vi "Autonomous Independent(2).vi"() -> ()   [LabVIEW 2014]
doc: "This VI is called when autonomous begins, and will automatically be terminated when autonomous ends. You can carry out timed or sensor driven robot movement independently without needing to return to the caller."
uses:
  <vilib>/Rock Robotics/WPI/Joystick/WPI_JoystickGetSetRefNum.vi
  <vilib>/Rock Robotics/Network Tables/SD Write Numeric Array.vi
  <vilib>/Rock Robotics/Network Tables/SD Read Number.vi
  <vilib>/Rock Robotics/WPI/RobotDrive/WPI_RobotDriveGetSetRefNum.vi
  <vilib>/Rock Robotics/WPI/RobotDrive/WPI_RobotDriveMecanumDrive_Cartesian.vi
  Robot Global Data.vi
panel:
  out "Current Movement, for debugging":T1 {"Z Joystick Value" scale=-1.0..1.0; "Y Joystick Value" scale=1.0..-1.0; "X Joystick Value" scale=-1.0..1.0}
  in  "Array of robot movements":T2(array[cluster]) {"Z Joystick Value" scale=-1.0..1.0; "Y Joystick Value" scale=1.0..-1.0; "X Joystick Value" scale=-1.0..1.0}
  # "Be sure to right-click and choose Data Operations>>Make Current Value default if you want to save the array values with the VI"
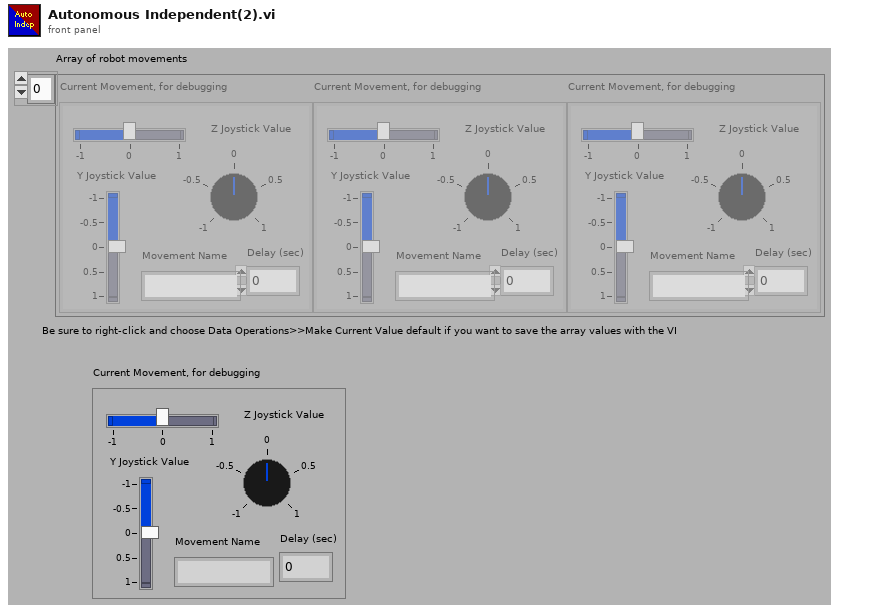
[diagram p1: front panel]
types:
  T1 = cluster{"X Joystick Value":dbl, "Y Joystick Value":dbl, "Z Joystick Value":dbl, "Delay (sec)":dbl, "Movement Name":string}
  T2 = cluster{"X Joystick Value":dbl, "Y Joystick Value":dbl, "Z Joystick Value":dbl, "Delay (sec)":dbl, "Movement Name":string}[]
  T3 = typedef "WPI_JoystickDevRef.ctl" = cluster{"Device":T4}
  T4 = typedef "WPI_JoystickDeviceEnum.ctl" = enum16{"USB 0", "USB 1", "USB 2", "USB 3", "USB 4", "USB 5"}
  T5 = typedef "WPI_EncoderDevRef.ctl" = cluster{"DevStatus":errorcluster, "EncoderIndex":T6, "CounterIndex":T7, "DistancePerCount":dbl, "Decoding Type":T8}
  T6 = typedef "FPGA_EncoderIdx.ctl" = enum8{"Enc 0", "Enc 1", "Enc 2", "Enc 3", "Enc 4", "Enc 5", "Enc 6", "Enc 7", "Invalid"}
  T7 = typedef "FPGA_CounterCtrSystemIndex.ctl" = enum8{"Ctr 0", "Ctr 1", "Ctr 2", "Ctr 3", "Ctr 4", "Ctr 5", "Ctr 6", "Ctr 7", "Invalid"}
  T8 = typedef "WPI_EncoderType.ctl" = enum16{"1x", "2x", "4x"}
  T9 = typedef "WPI_MotorControlDeviceRef.ctl" = cluster{"DeviceStatus":errorcluster, "Type":T10, "PWM":cluster{"Controller":T11, "PWM Channel":T12, "DeadBand":T13}, "CAN":cluster{"Device Number":u8, "Control Mode":T14, "Semaphore":T15, "Max Vout":dbl, "TalonSRX Control Mode":T16}, "Invert":bool, "TransformRef":T17, "InvTransformRef":T17}
  T10 = typedef "WPI_MotorControlType.ctl" = enum16{"PWM", "CAN", "CANTalonSRX"}
  T11 = typedef "FPGA_TypedefDigitalModule.ctl" = enum16{"Controller 1"}
  T12 = typedef "FPGA_DIOPWMChannel.ctl" = enum8{"PWM 0", "PWM 1", "PWM 2", "PWM 3", "PWM 4", "PWM 5", "PWM 6", "PWM 7", "PWM 8", "PWM 9", "PWM MXP 0", "PWM MXP 1", "PWM MXP 2", "PWM MXP 3", "PWM MXP 4", "PWM MXP 5", "PWM MXP 6", "PWM MXP 7", "PWM MXP 8", "PWM MXP 9", "Invalid"}
  T13 = typedef "WPI_PWMDeadband.ctl" = cluster{"Name":string, "maxPositivePwm":i32, "minPositivePwm":i32, "centerPwm":i32, "maxNegativePwm":i32, "minNegativePwm":i32, "angularRange":u16}
  T14 = typedef "WPI_CANJaguar_ControlMode.ctl" = enum8{"Percent VBus", "Current", "Speed", "Position", "Voltage"}
  T15 = typedef "Semaphore RefNum" = refnum<k1>
  T16 = typedef "WPI_CANTalonSRX_APIControlMode.ctl" = enum8{"Percent VBus", "Speed", "Position", "Slave", "Unchanged / Invalid"}
  T17 = typedef "WPI_PWMTransform_ConPane.ctl" = refnum<vi>
  T18 = typedef "WPI_RobotDriveDevRef.ctl" = cluster{"DevStatus":errorcluster, "Motors[]":T9[], "Square Inputs":bool, "Max Output":dbl}
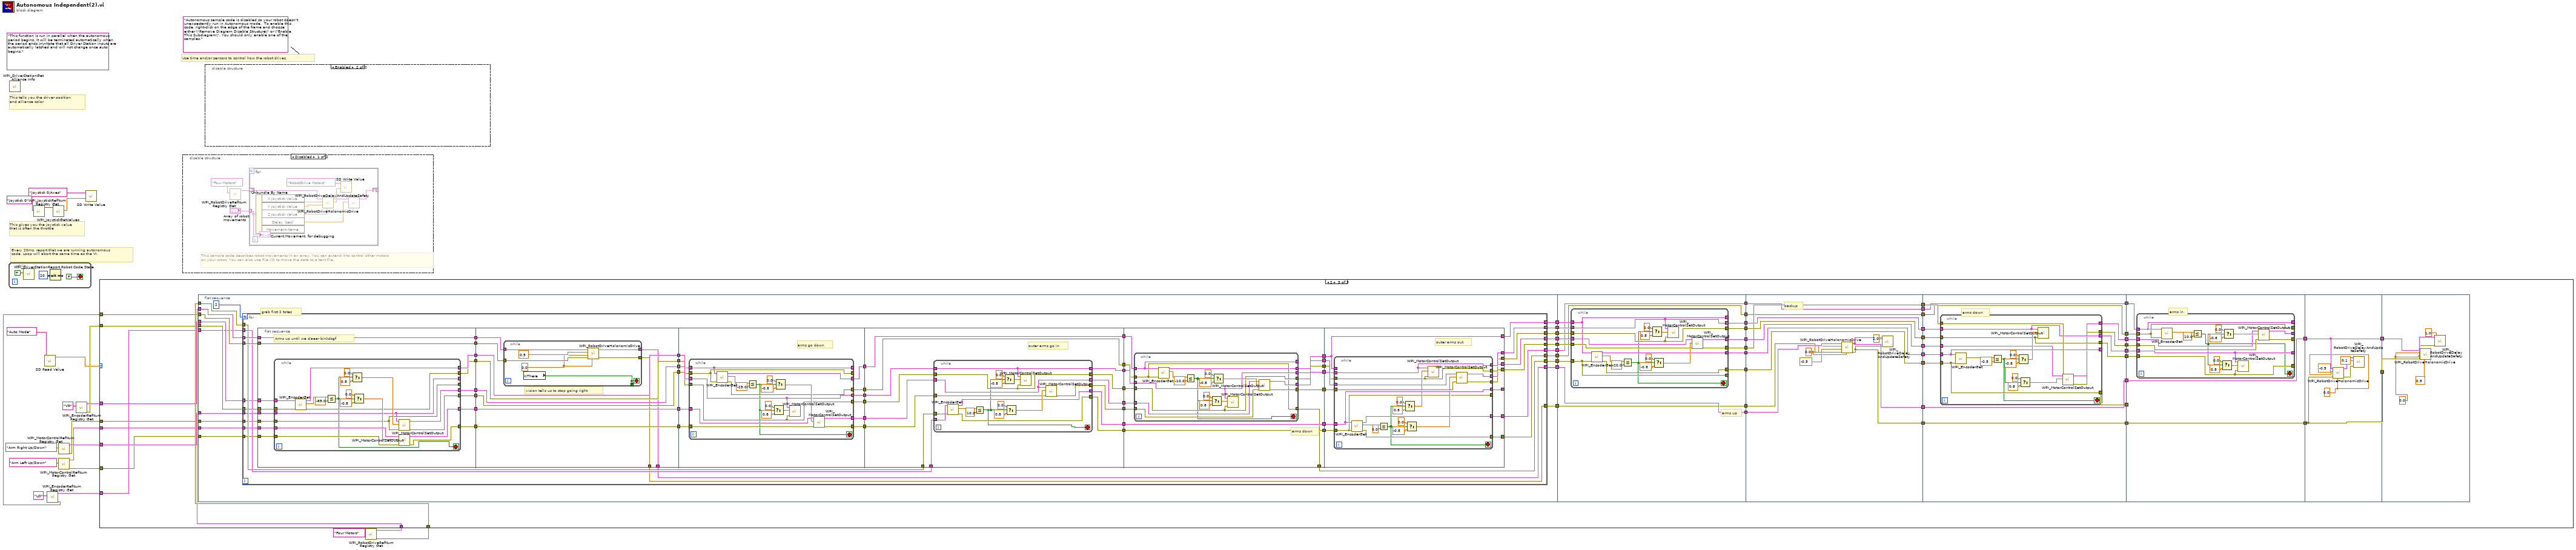
[diagram p0: block diagram]
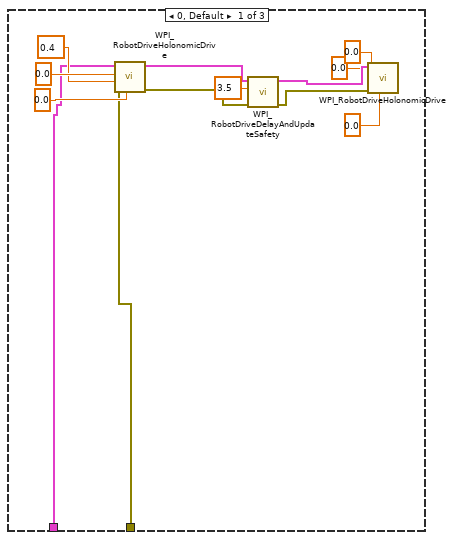
[diagram p2: hidden frame]
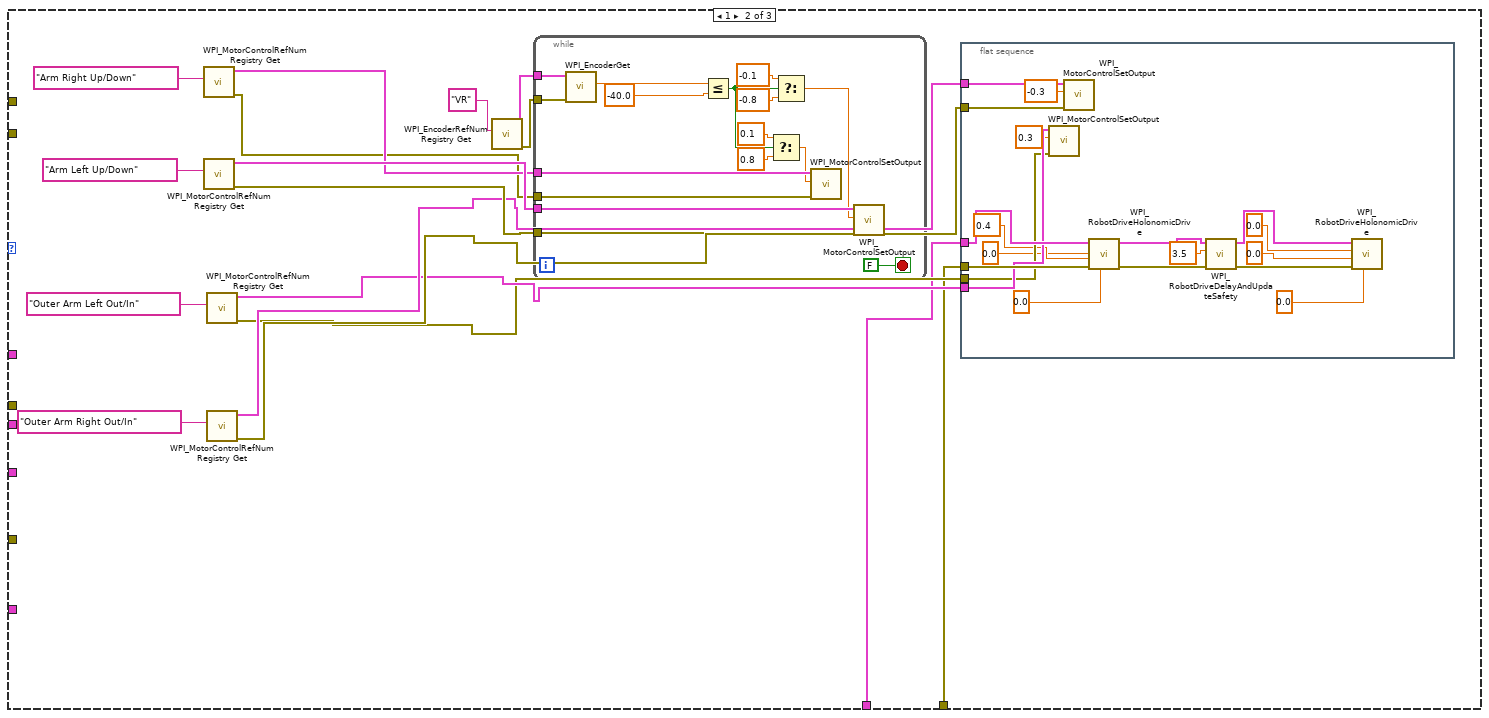
[diagram p3: hidden frame]
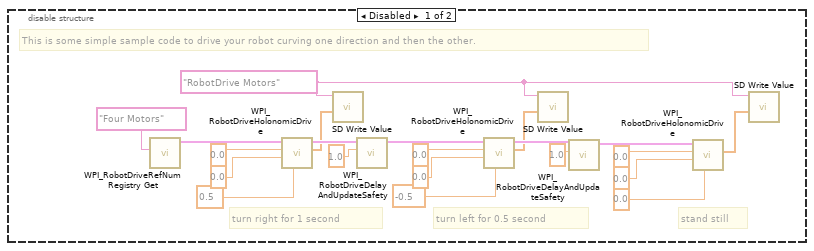
[diagram p5: hidden frame]
diagram:
  (unwired) "Autonomous sample code is disabled so your robot doesn't unexpectantly run in Autonomous mode.  To enable this code, right-click on the edge of the frame and choose either \"Remove Diagram Disable Structure\" or \"Enable This Subdiagram\". You should only enable one of the samples."
  (unwired) "This function is run in parallel when the autonomous period begins. It will be terminated automatically when the period ends.\n\nNote that all Driver Station inputs are automatically latched and will not change once auto begins."
  # "Every 20ms, report that we are running autonomous\ncode. Loop will abort the same time as the VI."
  # "This gives you the joystick value\nthat is often the throttle"
  # "Use time and/or sensors to control how the robot drives."
  # "This tells you the driver position\nand alliance color"
  n1 = while {
    stop <- FALSE stop-if-true
    n2 = call <vilib>:"WPI_DriverStationReport Robot Code State.vi"("Autonomous"=TRUE) -> ()  [unwired: 10 in, 1 out]
    n3 = Wait (ms)(milliseconds to wait=u32 20) -> ()  [unwired: 1 out]
  }
  n4 = call <vilib>:"WPI_DriverStationGet Alliance Info.vi"() -> ()  [unwired: 12 out]
  n5 = call <vilib>:"WPI_JoystickRefNum Registry Get.vi"("refnum name"="Joystick 0") -> ("JoystickDevRef"=w20:T3)  [unwired: 1 in, 9 out]
  n6 = call-poly <vilib>:"SD Read Value.vi"("Name"="Auto Mode") -> ("Numeric"=w17:dbl)  [unwired: 8 in, 2 out]
  n7 = call <vilib>:"WPI_EncoderRefNum Registry Get.vi"("refnum name"="LO") -> ("error out"=w1:errorcluster, "EncoderDevRef"=w2:T5)  [unwired: 9 in]
  n8 = call <vilib>:"WPI_JoystickGetValues.vi"("JoystickDevRef"=w20) -> ("Axes"=w18:dbl[])  [unwired: 6 in, 4 out]
  n9 = call <vilib>:"WPI_MotorControlRefNum Registry Get.vi"("refnum name"="Arm Right Up/Down") -> ("error out"=w5:errorcluster, "MotorControlDevRef"=w6:T9)  [unwired: 9 in]
  n10 = call <vilib>:"WPI_MotorControlRefNum Registry Get.vi"("refnum name"="Arm Left Up/Down") -> ("error out"=w3:errorcluster, "MotorControlDevRef"=w4:T9)  [unwired: 9 in]
  n11 = call <vilib>:"WPI_EncoderRefNum Registry Get.vi"("refnum name"="VR") -> ("error out"=w10:errorcluster, "EncoderDevRef"=w11:T5)  [unwired: 9 in]
  n12 = call-poly <vilib>:"SD Write Value.vi"("Numeric Array"=w18, "Name"="Joystick 0/Axes") -> ()  [unwired: 8 in, 2 out]
  n13 = disable-structure shown="Disabled" {
    frame Disabled {
      # "This sample code describes robot movements in an array. You can extend it to control other motors\non your robot. You can also use file I/O to move the data to a text file."
      n14 = call <vilib>:"WPI_RobotDriveRefNum Registry Get.vi"("refnum name"="Four Motors") -> ("RobotDriveDevRef"=w26:T18)  [unwired: 1 in, 9 out]
      n15 = for {
        shift-right: [w34] -> _
        shift-left: w26 -> [w35]
        tunnel: "Array of robot movements" -> [w30] mode=indexing
        n16 = Unbundle By Name(w30) -> ("X Joystick Value"=w33:dbl, "Y Joystick Value"=w32:dbl, "Z Joystick Value"=w29:dbl, "Delay (sec)"=w31:dbl)  [unwired: 1 out]
        n17 = call-poly <vilib>:"WPI_RobotDriveHolonomicDrive.vi"("Rotation"=w29, "Y"=w32, "X"=w33, "RobotDriveDevRef"=w35) -> ("Motor Values"=w28:dbl[], "RobotDriveDevRef"=w36:T18)  [unwired: 5 in, 1 out]
        n18 = call-poly <vilib>:"SD Write Value.vi"("Numeric Array"=w28, "Name"="RobotDrive Motors") -> ()  [unwired: 8 in, 2 out]
        n19 = call <vilib>:"WPI_RobotDriveDelayAndUpdateSafety.vi"("Delay (s)"=w31, "RobotDriveDevRef"=w36) -> ("RobotDriveDevRef 2"=w34:T18)  [unwired: 8 in, 1 out]
        "Current Movement, for debugging" <- w30
      }
    }
    frame Enabled {
    }
  }
  n20 = disable-structure shown="Enabled" {
    frame Disabled {
      w44 = "RobotDrive Motors" ("Name")
      # "This is some simple sample code to drive your robot curving one direction and then the other."
      # "stand still"
      # "turn left for 0.5 second"
      # "turn right for 1 second"
      n21 = call <vilib>:"WPI_RobotDriveRefNum Registry Get.vi"("refnum name"="Four Motors") -> ("RobotDriveDevRef"=w45:T18)  [unwired: 1 in, 9 out]
      n22 = call-poly <vilib>:"WPI_RobotDriveHolonomicDrive.vi"("Rotation"=0.5, "Y"=0.0 ("X axis value"), "X"=0.0 ("X axis value"), "RobotDriveDevRef"=w45) -> ("Motor Values"=w40:dbl[], "RobotDriveDevRef"=w52:T18)  [unwired: 5 in, 1 out]
      n23 = call-poly <vilib>:"SD Write Value.vi"("Numeric Array"=w40, "Name"=w44) -> ()  [unwired: 8 in, 2 out]
      n24 = call <vilib>:"WPI_RobotDriveDelayAndUpdateSafety.vi"("Delay (s)"=1.0, "RobotDriveDevRef"=w52) -> ("RobotDriveDevRef 2"=w51:T18)  [unwired: 8 in, 1 out]
      n25 = call-poly <vilib>:"WPI_RobotDriveHolonomicDrive.vi"("Rotation"=-0.5, "Y"=0.0 ("X axis value"), "X"=0.0 ("X axis value"), "RobotDriveDevRef"=w51) -> ("Motor Values"=w39:dbl[], "RobotDriveDevRef"=w50:T18)  [unwired: 5 in, 1 out]
      n26 = call-poly <vilib>:"SD Write Value.vi"("Numeric Array"=w39, "Name"=w44) -> ()  [unwired: 8 in, 2 out]
      n27 = call <vilib>:"WPI_RobotDriveDelayAndUpdateSafety.vi"("Delay (s)"=1.0, "RobotDriveDevRef"=w50) -> ("RobotDriveDevRef 2"=w49:T18)  [unwired: 8 in, 1 out]
      n28 = call-poly <vilib>:"WPI_RobotDriveHolonomicDrive.vi"("Rotation"=0.0 ("X axis value"), "Y"=0.0 ("X axis value"), "X"=0.0 ("X axis value"), "RobotDriveDevRef"=w49) -> ("Motor Values"=w38:dbl[])  [unwired: 5 in, 2 out]
      n29 = call-poly <vilib>:"SD Write Value.vi"("Numeric Array"=w38, "Name"=w44) -> ()  [unwired: 8 in, 2 out]
    }
    frame Enabled {
    }
  }
  n30 = call <vilib>:"WPI_RobotDriveRefNum Registry Get.vi"("refnum name"="Four Motors") -> ("error out"=w14:errorcluster, "RobotDriveDevRef"=w15:T18)  [unwired: 1 in, 8 out]
  n31 = case shown="2" w17 {
    tunnel: w15 -> [w60 w73 w133]
    tunnel: w14 -> [w59 w72 w132]
    tunnel: w11 -> [_ _ w131]
    tunnel: w10 -> [_ _ w130]
    tunnel: w6 -> [_ _ w129]
    tunnel: w5 -> [_ _ w128]
    tunnel: w4 -> [_ _ w127]
    tunnel: w3 -> [_ _ w126]
    tunnel: w2 -> [_ _ w125]
    tunnel: w1 -> [_ _ w124]
    frame 0, Default {
      n32 = call-poly <vilib>:"WPI_RobotDriveHolonomicDrive.vi"("Rotation"=0.0, "error in (no error)"=w59, "Y"=0.4 ("Magnitude"), "X"=0.0 ("Direction"), "RobotDriveDevRef"=w60) -> ("error out"=w69:errorcluster, "RobotDriveDevRef"=w68:T18)  [unwired: 4 in, 1 out]
      n33 = call <vilib>:"WPI_RobotDriveDelayAndUpdateSafety.vi"("error in (no error)"=w69, "Delay (s)"=3.5, "RobotDriveDevRef"=w68) -> ("error out"=w71:errorcluster, "RobotDriveDevRef 2"=w70:T18)  [unwired: 7 in]
      n34 = call-poly <vilib>:"WPI_RobotDriveHolonomicDrive.vi"("Rotation"=0.0, "error in (no error)"=w71, "Y"=0.0, "X"=0.0, "RobotDriveDevRef"=w70) -> ()  [unwired: 4 in, 3 out]
    }
    frame 1 {
      n35 = call <vilib>:"WPI_MotorControlRefNum Registry Get.vi"("refnum name"="Arm Right Up/Down") -> ("error out"=w81:errorcluster, "MotorControlDevRef"=w82:T9)  [unwired: 9 in]
      n36 = call <vilib>:"WPI_MotorControlRefNum Registry Get.vi"("refnum name"="Arm Left Up/Down") -> ("error out"=w84:errorcluster, "MotorControlDevRef"=w83:T9)  [unwired: 9 in]
      n37 = call <vilib>:"WPI_MotorControlRefNum Registry Get.vi"("refnum name"="Outer Arm Left Out/In") -> ("error out"=w74:errorcluster, "MotorControlDevRef"=w75:T9)  [unwired: 9 in]
      n38 = call <vilib>:"WPI_MotorControlRefNum Registry Get.vi"("refnum name"="Outer Arm Right Out/In") -> ("error out"=w76:errorcluster, "MotorControlDevRef"=w77:T9)  [unwired: 9 in]
      n39 = call <vilib>:"WPI_EncoderRefNum Registry Get.vi"("refnum name"="VR") -> ("error out"=w79:errorcluster, "EncoderDevRef"=w80:T5)  [unwired: 9 in]
      n40 = while {
        tunnel: w83 -> [w123]
        tunnel: w84 -> [w122]
        tunnel: w82 -> [w121]
        tunnel: w81 -> [w120]
        tunnel: w80 -> [w119]
        tunnel: w79 -> [w118]
        stop <- FALSE stop-if-true
        n41 = call <vilib>:"WPI_EncoderGet.vi"("error in (no error)"=w118, "EncoderDevRef"=w119) -> ("Distance"=w110:dbl)  [unwired: 4 in, 5 out]
        n42 = Less Or Equal?(x=w110, y=-40.0) -> (x <= y?=w116:bool)
        n43 = Select(t=0.1, s=w116, f=0.8 ("Output")) -> (s? t:f=w108:dbl)
        n44 = Select(t=-0.1, s=w116, f=-0.8 ("Output")) -> (s? t:f=w109:dbl)
        n45 = call <vilib>:"WPI_MotorControlSetOutput.vi"("error in (no error)"=w120, "Output"=w108, "MotorControlDevRef"=w121) -> ()  [unwired: 6 in, 3 out]
        n46 = call <vilib>:"WPI_MotorControlSetOutput.vi"("error in (no error)"=w122, "Output"=w109, "MotorControlDevRef"=w123) -> ()  [unwired: 6 in, 3 out]
      }
      n47 = flat-sequence {
        tunnel: w73 -> [w98]
        tunnel: w72 -> [w97]
        tunnel: w77 -> [w96]
        tunnel: w76 -> [w95]
        tunnel: w75 -> [w94]
        tunnel: w74 -> [w93]
        frame #0 {
          n48 = call <vilib>:"WPI_MotorControlSetOutput.vi"("error in (no error)"=w93, "Output"=0.3, "MotorControlDevRef"=w94) -> ()  [unwired: 6 in, 3 out]
          n49 = call <vilib>:"WPI_MotorControlSetOutput.vi"("error in (no error)"=w95, "Output"=-0.3, "MotorControlDevRef"=w96) -> ()  [unwired: 6 in, 3 out]
          n50 = call-poly <vilib>:"WPI_RobotDriveHolonomicDrive.vi"("Rotation"=0.0, "error in (no error)"=w97, "Y"=0.4 ("Magnitude"), "X"=0.0 ("Direction"), "RobotDriveDevRef"=w98) -> ("error out"=w105:errorcluster, "RobotDriveDevRef"=w106:T18)  [unwired: 4 in, 1 out]
          n51 = call <vilib>:"WPI_RobotDriveDelayAndUpdateSafety.vi"("error in (no error)"=w105, "Delay (s)"=3.5, "RobotDriveDevRef"=w106) -> ("error out"=w102:errorcluster, "RobotDriveDevRef 2"=w103:T18)  [unwired: 7 in]
          n52 = call-poly <vilib>:"WPI_RobotDriveHolonomicDrive.vi"("Rotation"=0.0, "error in (no error)"=w102, "Y"=0.0 ("Direction"), "X"=0.0 ("Magnitude"), "RobotDriveDevRef"=w103) -> ()  [unwired: 4 in, 3 out]
        }
      }
    }
    frame 2 {
      n53 = flat-sequence {
        tunnel: w133 -> [w197]
        tunnel: w124 -> [w196]
        tunnel: w129 -> [w195]
        tunnel: w128 -> [w194]
        tunnel: w131 -> [w193]
        tunnel: w130 -> [w192]
        tunnel: w127 -> [w191]
        tunnel: w126 -> [w190]
        tunnel: w125 -> [w189]
        tunnel: w132 -> [w188]
        tunnel: [w186] -> w176
        tunnel: [w185] -> w175
        tunnel: [w184] -> w174
        tunnel: [w183] -> w173
        tunnel: [w182] -> w172
        tunnel: [w181] -> w171
        tunnel: [w180] -> w170
        tunnel: [w179] -> w169
        tunnel: [w178] -> w168
        tunnel: [w177] -> w167
        tunnel: w176 -> [w448]
        tunnel: w175 -> [w447]
        tunnel: w174 -> [w446]
        tunnel: w173 -> [w445]
        tunnel: w172 -> [w444]
        tunnel: w171 -> [w443]
        tunnel: w170 -> [w442]
        tunnel: [w442] -> w166
        tunnel: [w441] -> w165
        tunnel: w169 -> [w441]
        tunnel: [w440] -> w164
        tunnel: [w439] -> w163
        tunnel: [w438] -> w162
        tunnel: [w437] -> w161
        tunnel: [w436] -> w160
        tunnel: [w435] -> w159
        tunnel: w168 -> [w434]
        tunnel: [w434] -> w158
        tunnel: [w433] -> w157
        tunnel: w167 -> [w433]
        tunnel: w166 -> [w482]
        tunnel: w165 -> [w481]
        tunnel: w164 -> [w480]
        tunnel: [w480] -> w156
        tunnel: [w479] -> w155
        tunnel: w163 -> [w479]
        tunnel: w162 -> [w478]
        tunnel: [w478] -> w154
        tunnel: [w477] -> w153
        tunnel: w161 -> [w477]
        tunnel: [w476] -> w152
        tunnel: w160 -> [w476]
        tunnel: [w475] -> w151
        tunnel: w159 -> [w475]
        tunnel: [w474] -> w150
        tunnel: w158 -> [w474]
        tunnel: w157 -> [w473]
        tunnel: [w473] -> w149
        tunnel: [w469] -> w148
        tunnel: [w468] -> w147
        tunnel: w156 -> [w497]
        tunnel: w155 -> [w496]
        tunnel: w154 -> [w495]
        tunnel: w153 -> [w494]
        tunnel: w152 -> [w493]
        tunnel: w151 -> [w492]
        tunnel: [w491] -> w146
        tunnel: w150 -> [w490]
        tunnel: [w490] -> w145
        tunnel: [w489] -> w144
        tunnel: w149 -> [w489]
        tunnel: [w488] -> w143
        tunnel: [w487] -> w142
        tunnel: [w486] -> w141
        tunnel: [w485] -> w140
        tunnel: w148 -> [w484]
        tunnel: [w484] -> w139
        tunnel: w147 -> [w483]
        tunnel: [w483] -> w138
        tunnel: w146 -> [_]
        tunnel: w145 -> [w522]
        tunnel: w144 -> [w521]
        tunnel: w143 -> [w520]
        tunnel: w142 -> [w519]
        tunnel: w141 -> [w518]
        tunnel: w140 -> [w517]
        tunnel: w139 -> [w516]
        tunnel: [w516] -> w137
        tunnel: w138 -> [w515]
        tunnel: [w515] -> w136
        tunnel: w137 -> [w546]
        tunnel: [w546] -> w135
        tunnel: w136 -> [w545]
        tunnel: [w545] -> w134
        tunnel: w135 -> [w551]
        tunnel: w134 -> [w550]
        frame #0 {
          # "grab first 2 totes"
          n54 = for {
            N: 2 -> [_]
            tunnel: w197 -> [w218]
            tunnel: w196 -> [w217]
            tunnel: w192 -> [w216]
            tunnel: w189 -> [w215]
            tunnel: w188 -> [w214]
            tunnel: w191 -> [w213]
            tunnel: w190 -> [w212]
            tunnel: w194 -> [w211]
            tunnel: w195 -> [w210]
            tunnel: w193 -> [w209]
            tunnel: [w208] -> w186
            tunnel: [w207] -> w185
            tunnel: [w205] -> w184
            tunnel: [w204] -> w183
            tunnel: [w203] -> w182
            tunnel: [w202] -> w181
            tunnel: [w201] -> w180
            tunnel: [w200] -> w179
            tunnel: [w199] -> w178
            tunnel: [w198] -> w177
            n55 = flat-sequence {
              tunnel: w217 -> [w265]
              tunnel: w218 -> [w266]
              tunnel: [w266] -> w252
              tunnel: [w265] -> w251
              tunnel: w216 -> [w264]
              tunnel: w213 -> [w263]
              tunnel: w212 -> [w262]
              tunnel: w210 -> [w253]
              tunnel: w211 -> [w261]
              tunnel: [w260] -> w250
              tunnel: [w259] -> w249
              tunnel: [w258] -> w248
              tunnel: [w257] -> w247
              tunnel: [w256] -> w246
              tunnel: [w255] -> w245
              tunnel: w209 -> [w254]
              tunnel: w252 -> [w297]
              tunnel: w251 -> [w296]
              tunnel: [w295] -> w244
              tunnel: w250 -> [w295]
              tunnel: [w294] -> w243
              tunnel: w249 -> [w294]
              tunnel: [w293] -> w242
              tunnel: w248 -> [w293]
              tunnel: [w292] -> w241
              tunnel: w247 -> [w292]
              tunnel: w246 -> [w291]
              tunnel: [w291] -> w240
              tunnel: [w290] -> w239
              tunnel: w245 -> [w290]
              tunnel: [w289] -> w201
              tunnel: [w288] -> w200
              tunnel: w244 -> [w316]
              tunnel: w243 -> [w315]
              tunnel: w242 -> [w314]
              tunnel: w241 -> [w313]
              tunnel: w240 -> [w312]
              tunnel: w239 -> [w311]
              tunnel: [w310] -> w238
              tunnel: [w309] -> w237
              tunnel: [w308] -> w236
              tunnel: [w307] -> w235
              tunnel: [w306] -> w234
              tunnel: [w305] -> w233
              tunnel: w215 -> [w349]
              tunnel: w214 -> [w348]
              tunnel: w238 -> [w347]
              tunnel: w237 -> [w346]
              tunnel: w236 -> [w345]
              tunnel: w235 -> [w344]
              tunnel: [w336] -> w232
              tunnel: [w343] -> w231
              tunnel: w234 -> [w342]
              tunnel: [w342] -> w230
              tunnel: [w341] -> w229
              tunnel: w233 -> [w341]
              tunnel: [w340] -> w228
              tunnel: [w339] -> w227
              tunnel: [w338] -> w226
              tunnel: [w337] -> w225
              tunnel: w232 -> [w381]
              tunnel: w231 -> [w380]
              tunnel: w230 -> [w379]
              tunnel: w229 -> [w378]
              tunnel: w228 -> [w377]
              tunnel: w227 -> [w376]
              tunnel: [w375] -> w224
              tunnel: w226 -> [w375]
              tunnel: w225 -> [w374]
              tunnel: [w374] -> w223
              tunnel: [w373] -> w222
              tunnel: [w372] -> w221
              tunnel: [w371] -> w220
              tunnel: [w370] -> w219
              tunnel: [w369] -> w206
              tunnel: [w368] -> w204
              tunnel: w224 -> [w413]
              tunnel: w223 -> [w412]
              tunnel: w222 -> [w411]
              tunnel: w221 -> [w410]
              tunnel: w220 -> [w409]
              tunnel: w219 -> [w408]
              tunnel: [w407] -> w208
              tunnel: [w406] -> w207
              tunnel: [w405] -> _
              tunnel: w206 -> [w404]
              tunnel: [w404] -> w205
              tunnel: [w403] -> w203
              tunnel: [w402] -> w202
              tunnel: [w401] -> w199
              tunnel: [w400] -> w198
              frame #0 {
                # "Arms up until we claear binkdsgf"
                n56 = while {
                  tunnel: w263 -> [w287]
                  tunnel: w262 -> [w286]
                  tunnel: [w274] -> _
                  tunnel: [w275] -> _
                  tunnel: w264 -> [w285]
                  tunnel: w254 -> [w276]
                  tunnel: w253 -> [w274]
                  tunnel: w261 -> [w275]
                  tunnel: [w273] -> w260
                  tunnel: [w272] -> w259
                  tunnel: [w271] -> w258
                  tunnel: [w270] -> w257
                  tunnel: [w269] -> w256
                  tunnel: [w268] -> w255
                  stop <- w267 stop-if-true
                  n57 = call <vilib>:"WPI_EncoderGet.vi"("error in (no error)"=w285, "EncoderDevRef"=w276) -> ("error out"=w268:errorcluster, "Distance"=w279:dbl, "EncoderDevRef"=w269:T5)  [unwired: 4 in, 3 out]
                  n58 = Less Or Equal?(x=w279, y=-85.0) -> (x <= y?=w267:bool)
                  n59 = Select(t=0.0, s=w267, f=0.8 ("Output")) -> (s? t:f=w277:dbl)
                  n60 = Select(t=0.0, s=w267, f=-0.8 ("Output")) -> (s? t:f=w278:dbl)
                  n61 = call <vilib>:"WPI_MotorControlSetOutput.vi"("error in (no error)"=w275, "Output"=w277, "MotorControlDevRef"=w274) -> ("error out"=w270:errorcluster, "MotorControlDevRef"=w271:T9)  [unwired: 6 in, 1 out]
                  n62 = call <vilib>:"WPI_MotorControlSetOutput.vi"("error in (no error)"=w286, "Output"=w278, "MotorControlDevRef"=w287) -> ("error out"=w272:errorcluster, "MotorControlDevRef"=w273:T9)  [unwired: 6 in, 1 out]
                }
              }
              frame #1 {
                # "vision tells us to stop going right"
                n63 = while {
                  tunnel: w297 -> [w304]
                  tunnel: w296 -> [w303]
                  tunnel: [w300] -> w289
                  tunnel: [w299] -> w288
                  tunnel: [w298] -> _
                  stop <- w298 stop-if-true
                  w301 = 0.0 ("Rotation")
                  n64 = global read "Robot Global Data.vi" "There"() -> (w298:bool)
                  n65 = call-poly <vilib>:"WPI_RobotDriveHolonomicDrive.vi"("Rotation"=w301, "error in (no error)"=w303, "Y"=w301, "X"=0.5, "RobotDriveDevRef"=w304) -> ("error out"=w299:errorcluster, "RobotDriveDevRef"=w300:T18)  [unwired: 4 in, 1 out]
                }
              }
              frame #2 {
                # "arms go down"
                n66 = while {
                  tunnel: w315 -> [w335]
                  tunnel: w314 -> [w325]
                  tunnel: w313 -> [w326]
                  tunnel: [w324] -> _
                  tunnel: [w325] -> w310
                  tunnel: [w326] -> w309
                  tunnel: w312 -> [w324]
                  tunnel: [w322] -> _
                  tunnel: w316 -> [w323]
                  tunnel: w311 -> [w322]
                  tunnel: [w321] -> w308
                  tunnel: [w320] -> w307
                  tunnel: [w319] -> w306
                  tunnel: [w318] -> w305
                  stop <- w317 stop-if-true
                  n67 = call <vilib>:"WPI_EncoderGet.vi"("error in (no error)"=w322, "EncoderDevRef"=w324) -> ("error out"=w318:errorcluster, "Distance"=w329:dbl, "EncoderDevRef"=w319:T5)  [unwired: 4 in, 3 out]
                  n68 = Less Or Equal?(x=w329, y=-25.0) -> (x <= y?=w317:bool)
                  n69 = Select(t=0.0, s=w317, f=0.8 ("Output")) -> (s? t:f=w327:dbl)
                  n70 = Select(t=0.0, s=w317, f=-0.8 ("Output")) -> (s? t:f=w328:dbl)
                  n71 = call <vilib>:"WPI_MotorControlSetOutput.vi"("error in (no error)"=w326, "Output"=w327, "MotorControlDevRef"=w325) -> ()  [unwired: 6 in, 3 out]
                  n72 = call <vilib>:"WPI_MotorControlSetOutput.vi"("error in (no error)"=w335, "Output"=w328, "MotorControlDevRef"=w323) -> ("error out"=w321:errorcluster, "MotorControlDevRef"=w320:T9)  [unwired: 6 in, 1 out]
                }
              }
              frame #3 {
                # "outer arms go in"
                n73 = while {
                  tunnel: [w359] -> w336
                  tunnel: [w358] -> w343
                  tunnel: [w354] -> w338
                  tunnel: [w352] -> w337
                  tunnel: [w356] -> w339
                  tunnel: w349 -> [w355]
                  tunnel: w348 -> [w353]
                  tunnel: w347 -> [w359]
                  tunnel: w346 -> [w358]
                  tunnel: w345 -> [w357]
                  tunnel: w344 -> [w356]
                  tunnel: [w351] -> w340
                  stop <- w350 stop-if-true
                  n74 = call <vilib>:"WPI_EncoderGet.vi"("error in (no error)"=w353, "EncoderDevRef"=w355) -> ("error out"=w352:errorcluster, "Distance"=w362:dbl, "EncoderDevRef"=w354:T5)  [unwired: 4 in, 3 out]
                  n75 = Less Or Equal?(x=w362, y=10.0) -> (x <= y?=w350:bool)
                  n76 = Select(t=0.0, s=w350, f=-0.8 ("Output")) -> (s? t:f=w360:dbl)
                  n77 = Select(t=0.0, s=w350, f=0.8 ("Output")) -> (s? t:f=w361:dbl)
                  n78 = call <vilib>:"WPI_MotorControlSetOutput.vi"("error in (no error)"=w358, "Output"=w360, "MotorControlDevRef"=w359) -> ()  [unwired: 6 in, 3 out]
                  n79 = call <vilib>:"WPI_MotorControlSetOutput.vi"("error in (no error)"=w357, "Output"=w361, "MotorControlDevRef"=w356) -> ("error out"=w351:errorcluster)  [unwired: 6 in, 2 out]
                }
              }
              frame #4 {
                # "arms down"
                n80 = while {
                  tunnel: w377 -> [w399]
                  tunnel: w381 -> [w389]
                  tunnel: w380 -> [w390]
                  tunnel: [w388] -> _
                  tunnel: [w389] -> w370
                  tunnel: [w390] -> w371
                  tunnel: w379 -> [w388]
                  tunnel: [w384] -> w368
                  tunnel: w376 -> [w387]
                  tunnel: [w386] -> w372
                  tunnel: [w385] -> w373
                  tunnel: w378 -> [w384]
                  tunnel: [w383] -> w369
                  stop <- w382 stop-if-true
                  n81 = call <vilib>:"WPI_EncoderGet.vi"("error in (no error)"=w384, "EncoderDevRef"=w388) -> ("Distance"=w393:dbl, "EncoderDevRef"=w383:T5)  [unwired: 4 in, 4 out]
                  n82 = Less Or Equal?(x=w393, y=-10.0) -> (x <= y?=w382:bool)
                  n83 = Select(t=0.0, s=w382, f=0.8 ("Output")) -> (s? t:f=w391:dbl)
                  n84 = Select(t=0.0, s=w382, f=-0.8 ("Output")) -> (s? t:f=w392:dbl)
                  n85 = call <vilib>:"WPI_MotorControlSetOutput.vi"("error in (no error)"=w390, "Output"=w391, "MotorControlDevRef"=w389) -> ()  [unwired: 6 in, 3 out]
                  n86 = call <vilib>:"WPI_MotorControlSetOutput.vi"("error in (no error)"=w399, "Output"=w392, "MotorControlDevRef"=w387) -> ("error out"=w386:errorcluster, "MotorControlDevRef"=w385:T9)  [unwired: 6 in, 1 out]
                }
              }
              frame #5 {
                # "outer arms out"
                n87 = while {
                  tunnel: w410 -> [w432]
                  tunnel: w408 -> [w414]
                  tunnel: w409 -> [w423]
                  tunnel: [w422] -> w405
                  tunnel: [w414] -> w407
                  tunnel: [w423] -> w406
                  tunnel: w413 -> [w422]
                  tunnel: [w418] -> _
                  tunnel: w411 -> [w421]
                  tunnel: [w420] -> w402
                  tunnel: [w419] -> w403
                  tunnel: w412 -> [w418]
                  tunnel: w404 -> [_]
                  tunnel: [w417] -> w401
                  tunnel: [w416] -> w400
                  stop <- w415 stop-if-true
                  n88 = call <vilib>:"WPI_EncoderGet.vi"("error in (no error)"=w418, "EncoderDevRef"=w422) -> ("error out"=w417:errorcluster, "Distance"=w426:dbl, "EncoderDevRef"=w416:T5)  [unwired: 4 in, 3 out]
                  n89 = Less Or Equal?(x=w426, y=0.0) -> (x <= y?=w415:bool)
                  n90 = Select(t=0.0, s=w415, f=0.8 ("Output")) -> (s? t:f=w424:dbl)
                  n91 = Select(t=0.0, s=w415, f=-0.8 ("Output")) -> (s? t:f=w425:dbl)
                  n92 = call <vilib>:"WPI_MotorControlSetOutput.vi"("error in (no error)"=w423, "Output"=w424, "MotorControlDevRef"=w414) -> ()  [unwired: 6 in, 3 out]
                  n93 = call <vilib>:"WPI_MotorControlSetOutput.vi"("error in (no error)"=w432, "Output"=w425, "MotorControlDevRef"=w421) -> ("error out"=w420:errorcluster, "MotorControlDevRef"=w419:T9)  [unwired: 6 in, 1 out]
                }
              }
            }
          }
        }
        frame #1 {
          # "arms up"
          n94 = while {
            tunnel: w443 -> [w467]
            tunnel: w448 -> [w457]
            tunnel: w447 -> [w458]
            tunnel: [w456] -> _
            tunnel: [w457] -> w440
            tunnel: [w458] -> w439
            tunnel: w446 -> [w456]
            tunnel: [w452] -> _
            tunnel: w444 -> [w455]
            tunnel: [w454] -> w435
            tunnel: [w453] -> w436
            tunnel: w445 -> [w452]
            tunnel: [w451] -> w438
            tunnel: [w450] -> w437
            stop <- w449 stop-if-true
            n95 = call <vilib>:"WPI_EncoderGet.vi"("error in (no error)"=w452, "EncoderDevRef"=w456) -> ("error out"=w450:errorcluster, "Distance"=w461:dbl, "EncoderDevRef"=w451:T5)  [unwired: 4 in, 3 out]
            n96 = Less Or Equal?(x=w461, y=-20.0) -> (x <= y?=w449:bool)
            n97 = Select(t=0.0, s=w449, f=0.8 ("Output")) -> (s? t:f=w459:dbl)
            n98 = Select(t=0.0, s=w449, f=-0.8 ("Output")) -> (s? t:f=w460:dbl)
            n99 = call <vilib>:"WPI_MotorControlSetOutput.vi"("error in (no error)"=w458, "Output"=w459, "MotorControlDevRef"=w457) -> ()  [unwired: 6 in, 3 out]
            n100 = call <vilib>:"WPI_MotorControlSetOutput.vi"("error in (no error)"=w467, "Output"=w460, "MotorControlDevRef"=w455) -> ("error out"=w454:errorcluster, "MotorControlDevRef"=w453:T9)  [unwired: 6 in, 1 out]
          }
        }
        frame #2 {
          w471 = 0.0 ("Rotation")
          # "backup"
          n101 = call-poly <vilib>:"WPI_RobotDriveHolonomicDrive.vi"("Rotation"=w471, "error in (no error)"=w481, "Y"=-0.5 ("X"), "X"=w471, "RobotDriveDevRef"=w482) -> ("error out"=w468:errorcluster, "RobotDriveDevRef"=w469:T18)  [unwired: 4 in, 1 out]
          n102 = call <vilib>:"WPI_RobotDriveDelayAndUpdateSafety.vi"("error in (no error)"=w468, "Delay (s)"=2.0, "RobotDriveDevRef"=w469) -> ()  [unwired: 7 in, 2 out]
        }
        frame #3 {
          # "arms down"
          n103 = while {
            tunnel: w492 -> [w514]
            tunnel: w497 -> [w504]
            tunnel: w496 -> [w505]
            tunnel: [w503] -> _
            tunnel: [w504] -> w488
            tunnel: [w505] -> w487
            tunnel: w495 -> [w503]
            tunnel: [w499] -> w491
            tunnel: w493 -> [w502]
            tunnel: [w501] -> w485
            tunnel: [w500] -> w486
            tunnel: w494 -> [w499]
            stop <- w498 stop-if-true
            n104 = call <vilib>:"WPI_EncoderGet.vi"("error in (no error)"=w499, "EncoderDevRef"=w503) -> ("Distance"=w508:dbl)  [unwired: 4 in, 5 out]
            n105 = Less Or Equal?(x=w508, y=-0.5) -> (x <= y?=w498:bool)
            n106 = Select(t=0.0, s=w498, f=-0.8 ("Output")) -> (s? t:f=w506:dbl)
            n107 = Select(t=0.0, s=w498, f=0.8 ("Output")) -> (s? t:f=w507:dbl)
            n108 = call <vilib>:"WPI_MotorControlSetOutput.vi"("error in (no error)"=w505, "Output"=w506, "MotorControlDevRef"=w504) -> ()  [unwired: 6 in, 3 out]
            n109 = call <vilib>:"WPI_MotorControlSetOutput.vi"("error in (no error)"=w514, "Output"=w507, "MotorControlDevRef"=w502) -> ("error out"=w501:errorcluster, "MotorControlDevRef"=w500:T9)  [unwired: 6 in, 1 out]
          }
        }
        frame #4 {
          # "arms in"
          n110 = while {
            tunnel: w517 -> [w539]
            tunnel: w520 -> [w529]
            tunnel: w519 -> [w530]
            tunnel: [w528] -> _
            tunnel: [w529] -> _
            tunnel: [w530] -> _
            tunnel: w521 -> [w528]
            tunnel: [w524] -> _
            tunnel: w518 -> [w527]
            tunnel: [w526] -> _
            tunnel: [w525] -> _
            tunnel: w522 -> [w524]
            stop <- w523 stop-if-true
            n111 = call <vilib>:"WPI_EncoderGet.vi"("error in (no error)"=w524, "EncoderDevRef"=w528) -> ("Distance"=w533:dbl)  [unwired: 4 in, 5 out]
            n112 = Less Or Equal?(x=w533, y=10.0) -> (x <= y?=w523:bool)
            n113 = Select(t=0.0, s=w523, f=0.8 ("Output")) -> (s? t:f=w531:dbl)
            n114 = Select(t=0.0, s=w523, f=-0.8 ("Output")) -> (s? t:f=w532:dbl)
            n115 = call <vilib>:"WPI_MotorControlSetOutput.vi"("error in (no error)"=w530, "Output"=w531, "MotorControlDevRef"=w529) -> ()  [unwired: 6 in, 3 out]
            n116 = call <vilib>:"WPI_MotorControlSetOutput.vi"("error in (no error)"=w539, "Output"=w532, "MotorControlDevRef"=w527) -> ("error out"=w526:errorcluster, "MotorControlDevRef"=w525:T9)  [unwired: 6 in, 1 out]
          }
        }
        frame #5 {
          w540 = 0.0 ("Rotation")
          n117 = call-poly <vilib>:"WPI_RobotDriveHolonomicDrive.vi"("Rotation"=w540, "error in (no error)"=w545, "Y"=-0.5, "X"=w540, "RobotDriveDevRef"=w546) -> ("error out"=w542:errorcluster, "RobotDriveDevRef"=w543:T18)  [unwired: 4 in, 1 out]
          n118 = call <vilib>:"WPI_RobotDriveDelayAndUpdateSafety.vi"("error in (no error)"=w542, "Delay (s)"=0.1, "RobotDriveDevRef"=w543) -> ()  [unwired: 7 in, 2 out]
        }
        frame #6 {
          w547 = 0.0 ("Rotation")
          n119 = call-poly <vilib>:"WPI_RobotDriveHolonomicDrive.vi"("Rotation"=0.5, "error in (no error)"=w550, "Y"=w547, "X"=w547, "RobotDriveDevRef"=w551) -> ("error out"=w552:errorcluster, "RobotDriveDevRef"=w553:T18)  [unwired: 4 in, 1 out]
          n120 = call <vilib>:"WPI_RobotDriveDelayAndUpdateSafety.vi"("error in (no error)"=w552, "Delay (s)"=1.0, "RobotDriveDevRef"=w553) -> ()  [unwired: 7 in, 2 out]
        }
      }
    }
  }
